vi "createADCOffsetSensitivityFrame.vi"(8 "error in (no error)":errorcluster, 9 "TriggerIRQ":bool, 10 "WaitForTrigger":bool, 11 "ILC in":refnum<class "ILC.lvclass">) -> (0 "error out":errorcluster, 2 "Frame":T1 {"Data" format="%02x"}, 3 "ILC out":refnum<class "ILC.lvclass">)   [LabVIEW 2015, in "RTILC.lvlib" / "ILC.lvclass"]
uses:
  ILC.lvclass
  Common_RT_Modbus/DataTypes/Frame.ctl
  Common_RT_Modbus/DynamicFrameBuilder/DynamicFrameBuilder.lvclass
  ILC.lvclass/ILC.ctl
  Common_RT_Modbus/RTModbus.lvlib
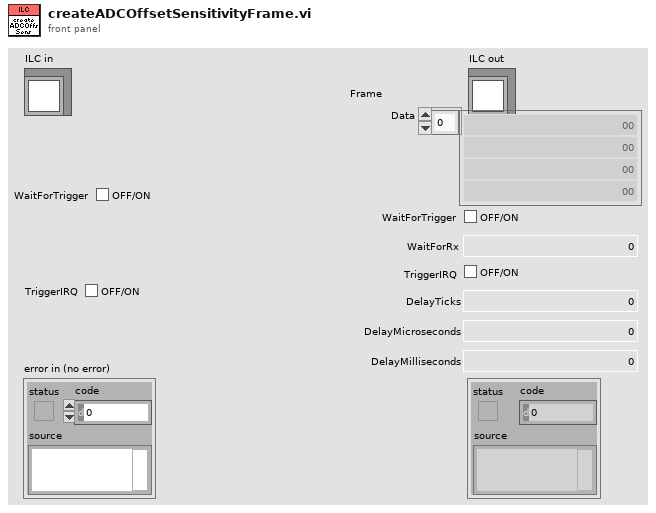
[diagram p1: front panel]
types:
  T1 = typedef "RTModbus.lvlib/Frame.ctl" = cluster{"Data":u8[], "WaitForTrigger":bool, "WaitForRx":u16, "TriggerIRQ":bool, "DelayTicks":u16, "DelayMicroseconds":u16, "DelayMilliseconds":u16}
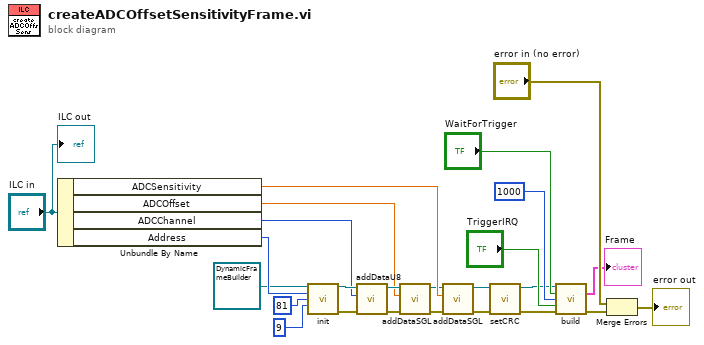
[diagram p0: block diagram]
diagram:
  n1 = Unbundle By Name("ILC in") -> ("ADCSensitivity"=w5:sgl, "ADCOffset"=w8:sgl, "ADCChannel"=w6:u8, "Address"=w21:u8)
  n2 = call "init.vi"("DynamicFrameBuilder in"=refnum<class "DynamicFrameBuilder.lvclass"> refnum ("RTModbus.lvlib:DynamicFrameBuilder.lvclass"), "Address"=w21, "Function"=u8 81, "DataSize"=9) -> ("DynamicFrameBuilder out"=w19:refnum<class "DynamicFrameBuilder.lvclass">, "error out"=w18:errorcluster)  [unwired: 10 in]
  n3 = call "addDataU8.vi"("error in (no error)"=w18, "Data"=w6, "DynamicFrameBuilder in"=w19) -> ("error out"=w7:errorcluster, "DynamicFrameBuilder out"=w9:refnum<class "DynamicFrameBuilder.lvclass">)  [unwired: 7 in]
  n4 = call "addDataSGL.vi"("error in (no error)"=w7, "Data"=w8, "DynamicFrameBuilder in"=w9) -> ("error out"=w3:errorcluster, "DynamicFrameBuilder out"=w4:refnum<class "DynamicFrameBuilder.lvclass">)  [unwired: 7 in]
  n5 = call "addDataSGL.vi"("error in (no error)"=w3, "Data"=w5, "DynamicFrameBuilder in"=w4) -> ("error out"=w2:errorcluster, "DynamicFrameBuilder out"=w1:refnum<class "DynamicFrameBuilder.lvclass">)  [unwired: 7 in]
  n6 = call "setCRC.vi"("error in (no error)"=w2, "DynamicFrameBuilder in"=w1) -> ("error out"=w17:errorcluster, "DynamicFrameBuilder out"=w11:refnum<class "DynamicFrameBuilder.lvclass">)  [unwired: 8 in]
  n7 = call "build.vi"("DynamicFrameBuilder in"=w11, "WaitForTrigger"="WaitForTrigger", "WaitForRxTimeout"=u16 1000, "TriggerIRQ"="TriggerIRQ", "error in (no error)"=w17) -> ("Frame"=→"Frame":T1, "error out"=w12:errorcluster)  [unwired: 8 in, 1 out]
  n8 = Merge Errors("error in (no error)", w12) -> (→"error out":errorcluster)
  "ILC out" <- "ILC in"
